vi "Set Home.vi"(8 "error in (no error)":errorcluster, 11 "Stage Controller in":refnum<class "Stage Controller.lvclass">) -> (0 "error out":errorcluster, 3 "Stage Controller out":refnum<class "Stage Controller.lvclass">)   [LabVIEW 2018, in "Stage Controller.lvlib" / "Stage Controller.lvclass"]
uses:
  Stage Controller.lvclass
  Stage Controller.lvclass/Stage Controller.ctl
  Resources/GLOBAL/GLOBAL Debug.vi
  Microscope/ti2lv/ti2lv.lvlib
  <instrlib>/ASI TG-1000/ASI TG-1000.lvlib
  Stage Controller.lvlib
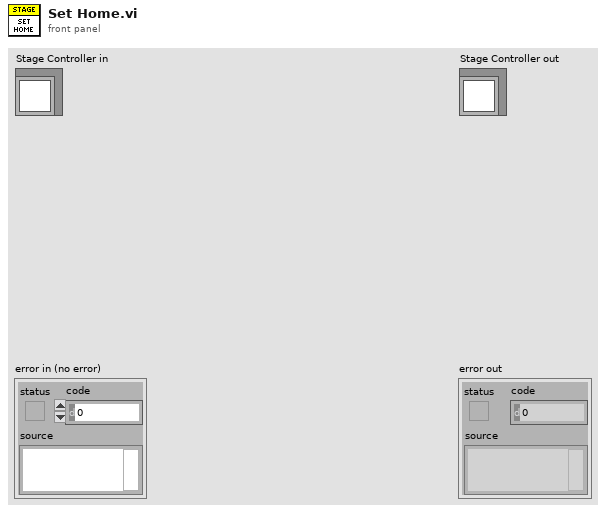
[diagram p1: front panel]
types:
  T1 = enum16{"Disabled", "ESP301", "Ti2", "Ludl", "ASI"}
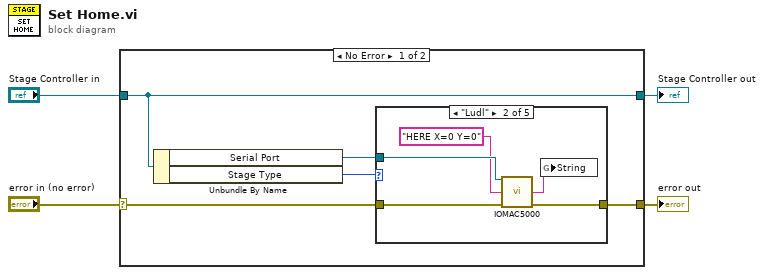
[diagram p0: block diagram]
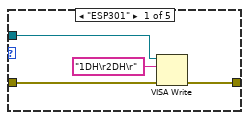
[diagram p2: hidden frame]
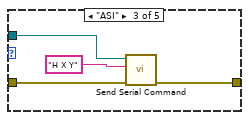
[diagram p3: hidden frame]
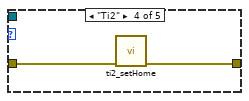
[diagram p4: hidden frame]
diagram:
  n1 = case shown="No Error" "error in (no error)" {
    selector: "error in (no error)" -> [w8 w27]
    tunnel: [w7 w27] -> w3
    tunnel: [w9 w26] -> w1
    tunnel: "Stage Controller in" -> [w9 w26]
    frame No Error {
      n2 = Unbundle By Name(w9) -> ("Serial Port"=w6:refnum<visa-resource-name>, "Stage Type"=w5:T1)
      n3 = case shown="\"Ludl\"" w5 {
        tunnel: w8 -> [w11 w17 w22 w24 w25]
        tunnel: [w12 w18 w19 w23 w25] -> w7
        tunnel: w6 -> [w10 w16 w21 _ _]
        frame "ESP301" {
          n4 = VISA Write(VISA resource name=w10, write buffer="1DH\r2DH\r", error in (no error)=w11) -> (error out=w12:errorcluster)  [unwired: 2 out]
        }
        frame "Ludl" {
          n5 = call "IOMAC5000.vi"("VISA  IN"=w16, "Command (to ctlr)"="HERE X=0 Y=0" ("true string"), "error in"=w17) -> ("Raw Response"=w14:string, "error out"=w18:errorcluster)  [unwired: 9 in, 2 out]
          n6 = global write "GLOBAL Debug.vi" "String"(w14) -> ()
        }
        frame "ASI" {
          n7 = call <instrlib>:"Send Serial Command.vi"("error in (no error)"=w22, "Command"="H X Y", "VISA in"=w21) -> ("error out"=w19:errorcluster)  [unwired: 6 in, 2 out]
        }
        frame "Ti2" {
          n8 = call "ti2_setHome.vi"("error in (no error)"=w24) -> ("error out"=w23:errorcluster)  [unwired: 10 in]
        }
        frame "Disabled", Default {
        }
      }
    }
    frame Error {
    }
  }
  "error out" <- w3
  "Stage Controller out" <- w1
